vi "Raise Out of Range Error.vi"(0 "Parameter Name":string, 5 "Upper Limit":string, 7 "Lower Limit":string, 9 "As Found":string, 11 "error in (no error)":errorcluster) -> (15 "error out":errorcluster)   [LabVIEW 2018, in "MIPI RFFE API.lvlib"]
uses:
  MIPI RFFE API.lvlib
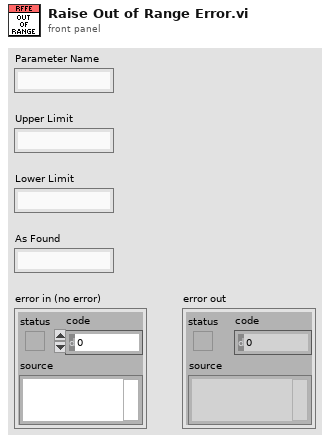
[diagram p1: front panel]
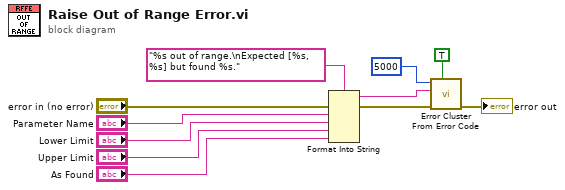
[diagram p0: block diagram]
diagram:
  n1 = Format Into String(format string="%s out of range.\nExpected [%s, %s] but found %s." ("initial string"), error in="error in (no error)", "Parameter Name", "Lower Limit", "Upper Limit", "As Found") -> (resulting string=w5:string, error out=w1:errorcluster)  [unwired: 1 in]
  n2 = call <vilib>:"Error Cluster From Error Code.vi"("show call chain? (False)"=TRUE, "error in (no error)"=w1, "error message (\"\")"=w5, "error code (0)"=5000) -> ("error out"=→"error out":errorcluster)  [unwired: 5 in]
